vi "Calibration_Read_streaming_3s.vi"(8 "error in (no error)":errorcluster, 11 "USB":tag) -> (0 "error out":errorcluster, 2 "uABank1":dbl)   [LabVIEW 2015]
uses:
  <vilib>/DAQmx/read.llb/DAQmx Read (Analog Wfm 1Chan NSamp).vi
  <vilib>/DAQmx/miscellaneous.llb/DAQmx Fill In Error Info.vi
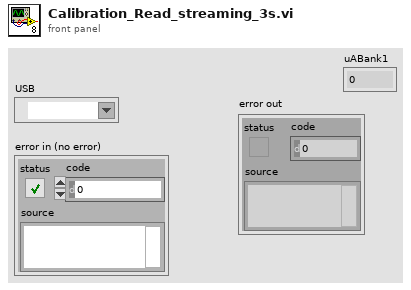
[diagram p1: front panel]
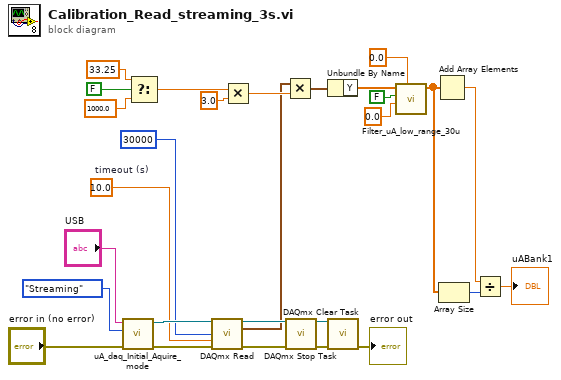
[diagram p0: block diagram]
diagram:
  w26 = 10.0  # timeout (s)
  n1 = call "uA_daq_Initial_Aquire_mode.vi"("error in"="error in (no error)", "Acquire Mode"=enum16{"Streaming", "Read All", "Stop"}."Streaming", "USB DAQ"="USB") -> ("error out"=w22:errorcluster, "Refnum out"=w28:refnum<k21>)  [unwired: 7 in]
  n2 = Select(t=sgl 33.25 ("y"), s=FALSE, f=sgl 1000.0 ("y")) -> (s? t:f=w12:sgl)
  n3 = call-poly <vilib>:"DAQmx Read.vi"("task/channels in"=w28, "number of samples per channel"=30000, "timeout"=w26, "error in"=w22) -> ("task out"=w19:refnum<k21>, "data"=w8:waveform(dbl), "error out"=w17:errorcluster)  [unwired: 9 in]
  n4 = Multiply(x=w12, y=sgl 3.0) -> (x*y=w9:sgl)
  n5 = Multiply(x=w8, y=w9) -> (x*y=w7:waveform(dbl))
  n6 = call <vilib>:"DAQmx Stop Task.vi"("task/channels in"=w19, "error in"=w17) -> ("task out"=w18:refnum<k21>, "error out"=w15:errorcluster)  [unwired: 12 in]
  n7 = Unbundle By Name(w7) -> ("Y"=w5:dbl[])
  n8 = call <vilib>:"DAQmx Clear Task.vi"("task in"=w18, "error in"=w15) -> ("error out"=→"error out":errorcluster)  [unwired: 13 in]
  n9 = call "Filter_uA_low_range_30u.vi"("Frequency"=0.0, "uA_calib_0"=0.0, "mA/uA"=FALSE, "in"=w5) -> ("out"=w4:dbl[])  [unwired: 7 in]
  n10 = Add Array Elements(numeric array=w4) -> (sum=w21:dbl)
  n11 = Array Size(array=w4) -> (size(s)=w20:i32)
  n12 = Divide(x=w21, y=w20) -> (x/y=→"uABank1":dbl)
